vi "Servo.vi"() -> ()   [LabVIEW 2013]
uses:
  <vilib>/Rock Robotics/SystemInterfaces/DIO/FPGA_DIOPWMChannel.ctl
panel:
  in  "State Select":enum16{"Open", "Run", "End"}(ring)
  in  "Shoot Frisby?":bool
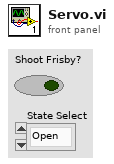
[diagram p1: front panel]
types:
  T1 = typedef "FPGA_DIOPWMChannel.ctl" = enum8{"PWM 1", "PWM 2", "PWM 3", "PWM 4", "PWM 5", "PWM 6", "PWM 7", "PWM 8", "PWM 9", "PWM 10", "Invalid"}
  T2 = typedef "WPI_ServoDeviceRef.ctl" = cluster{"DeviceStatus":errorcluster, "Digital Module":T3, "PWM Channel":T1, "DeadBand":T4}
  T3 = typedef "FPGA_TypedefDigitalModule.ctl" = enum16{"Digital Module 1", "Digital Module 2"}
  T4 = typedef "WPI_PWMDeadband.ctl" = cluster{"Name":string, "maxPositivePwm":i32, "minPositivePwm":i32, "centerPwm":i32, "maxNegativePwm":i32, "minNegativePwm":i32, "angularRange":u16}
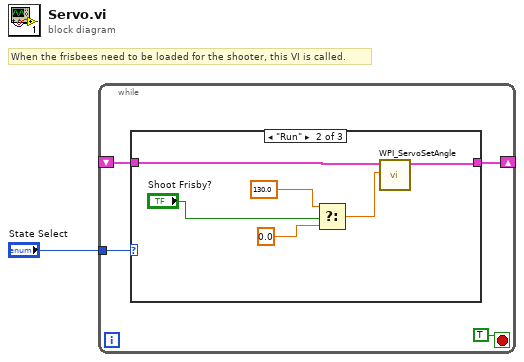
[diagram p0: block diagram]
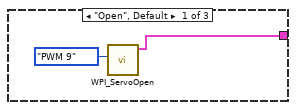
[diagram p2: hidden frame]
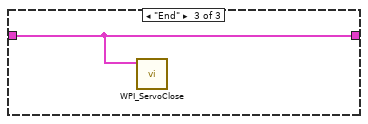
[diagram p3: hidden frame]
diagram:
  # "When the frisbees need to be loaded for the shooter, this VI is called."
  n1 = while {
    tunnel: "State Select" -> [w5]
    shift-right: [w4] -> _
    shift-left: _ -> [w3]
    stop <- TRUE stop-if-true
    n2 = case shown="\"Run\"" w5 {
      tunnel: [w6 w10 w14] -> w4
      tunnel: w3 -> [_ w9 w14]
      frame "Open", Default {
        n3 = call <vilib>:"WPI_ServoOpen.vi"("PWM Channel"=FPGA_DIOPWMChannel."PWM 9") -> ("ServoDeviceRef"=w6:T2)  [unwired: 9 in, 1 out]
      }
      frame "Run" {
        n4 = Select(t=130.0, s="Shoot Frisby?", f=0.0) -> (s? t:f=w11:dbl)
        n5 = call <vilib>:"WPI_ServoSetAngle.vi"("Angle"=w11, "ServoDeviceRef"=w9) -> ("ServoDeviceRef"=w10:T2)  [unwired: 8 in, 1 out]
      }
      frame "End" {
        n6 = call <vilib>:"WPI_ServoClose.vi"("MotorControlDevRef"=w14) -> ()  [unwired: 10 in, 1 out]
      }
    }
  }
